vi "Emballge_BDD_Lecture_balises_PPXml_V2.vi"(8 "entrée d'erreur (pas d'erreur)":errorcluster, 11 "appended path":path) -> (0 "sortie d'erreur":errorcluster, 1 "Nb_valve_par_carton":string, 3 "affiche_code_barre_client":string, 4 "melange_des_lots_possible":string, 5 "Code_Barre_Fixe":string, 7 "Indice":string)   [LabVIEW 2020]
uses:
  <vilib>/xml/Load XML File.vi
  <vilib>/xml/Close Reference(Node).vi
  <vilib>/xml/NI_XML.lvlib
panel:
  out "x-y":u32
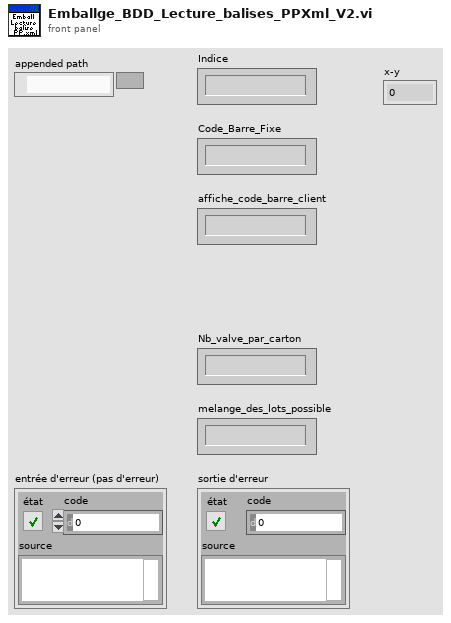
[diagram p1: front panel]
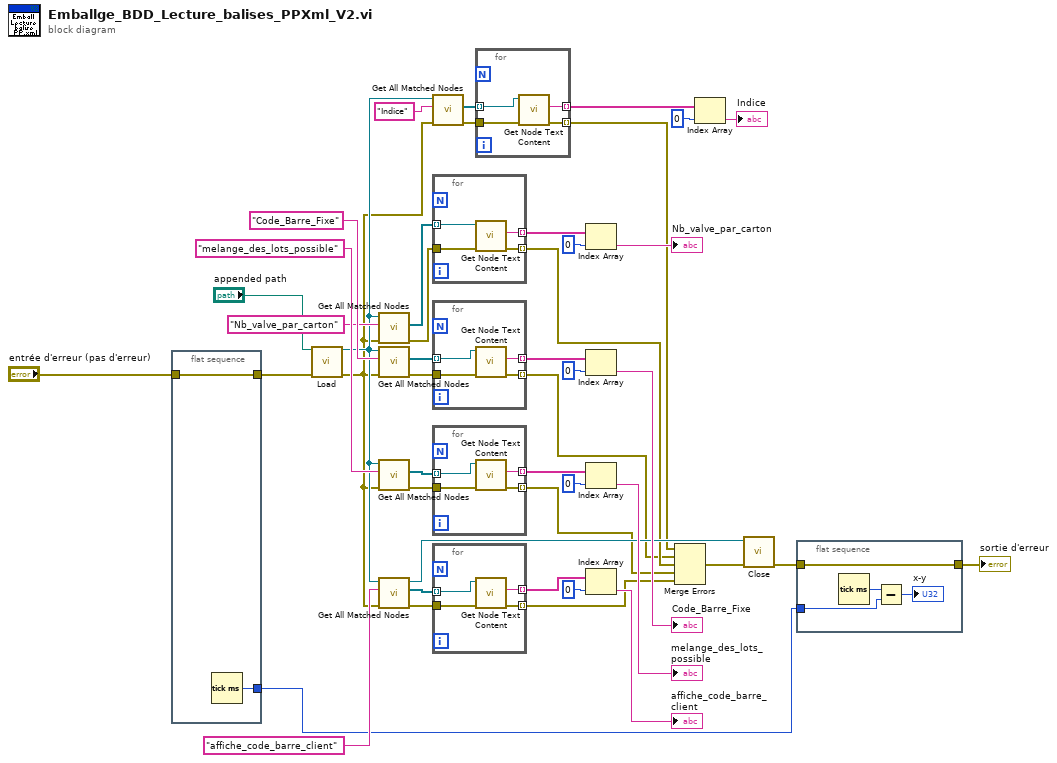
[diagram p0: block diagram]
diagram:
  n1 = flat-sequence {
    tunnel: [w47] -> w33
    tunnel: "entrée d'erreur (pas d'erreur)" -> [w47]
    tunnel: [w46] -> w30
    frame #0 {
      n2 = Tick Count (ms)() -> (millisecond timer value=w46:u32)
    }
  }
  n3 = call-poly <vilib>:"Load.vi"("path to XML document"="appended path", "error in (no error)"=w33) -> ("DOM document out"=w6:refnum<k20>, "error out"=w5:errorcluster)  [unwired: 11 in, 1 out]
  n4 = call <vilib>:"Get All Matched Nodes.vi"("error in (no error)"=w5, "XPath expression"="Nb_valve_par_carton", "node in"=w6) -> ("error out"=w20:errorcluster, "node result array"=w21:refnum<k20>[])  [unwired: 6 in, 1 out]
  n5 = call <vilib>:"Get All Matched Nodes.vi"("error in (no error)"=w5, "XPath expression"="Code_Barre_Fixe", "node in"=w6) -> ("error out"=w24:errorcluster, "node result array"=w25:refnum<k20>[])  [unwired: 6 in, 1 out]
  n6 = call <vilib>:"Get All Matched Nodes.vi"("error in (no error)"=w5, "XPath expression"="melange_des_lots_possible", "node in"=w6) -> ("error out"=w16:errorcluster, "node result array"=w17:refnum<k20>[])  [unwired: 6 in, 1 out]
  n7 = call <vilib>:"Get All Matched Nodes.vi"("error in (no error)"=w5, "XPath expression"="affiche_code_barre_client", "node in"=w6) -> ("error out"=w12:errorcluster, "node result array"=w13:refnum<k20>[], "node out"=w7:refnum<k20>)  [unwired: 6 in]
  n8 = call <vilib>:"Get All Matched Nodes.vi"("error in (no error)"=w5, "XPath expression"="Indice", "node in"=w6) -> ("error out"=w27:errorcluster, "node result array"=w28:refnum<k20>[])  [unwired: 6 in, 1 out]
  n9 = for {
    tunnel: w21 -> [w51] mode=indexing
    tunnel: w20 -> [w50]
    tunnel: [w49] -> w3 mode=indexing
    tunnel: [w48] -> w18 mode=indexing
    n10 = call <vilib>:"Get Node Text Content.vi"("error in (no error)"=w50, "node in"=w51) -> ("error out"=w49:errorcluster, "node text"=w48:string)  [unwired: 7 in, 1 out]
  }
  n11 = for {
    tunnel: w25 -> [w55] mode=indexing
    tunnel: w24 -> [w54]
    tunnel: [w53] -> w2 mode=indexing
    tunnel: [w52] -> w22 mode=indexing
    n12 = call <vilib>:"Get Node Text Content.vi"("error in (no error)"=w54, "node in"=w55) -> ("error out"=w53:errorcluster, "node text"=w52:string)  [unwired: 7 in, 1 out]
  }
  n13 = for {
    tunnel: w17 -> [w59] mode=indexing
    tunnel: w16 -> [w58]
    tunnel: [w57] -> w4 mode=indexing
    tunnel: [w56] -> w14 mode=indexing
    n14 = call <vilib>:"Get Node Text Content.vi"("error in (no error)"=w58, "node in"=w59) -> ("error out"=w57:errorcluster, "node text"=w56:string)  [unwired: 7 in, 1 out]
  }
  n15 = for {
    tunnel: w13 -> [w63] mode=indexing
    tunnel: w12 -> [w62]
    tunnel: [w61] -> w10 mode=indexing
    tunnel: [w60] -> w9 mode=indexing
    n16 = call <vilib>:"Get Node Text Content.vi"("error in (no error)"=w62, "node in"=w63) -> ("error out"=w61:errorcluster, "node text"=w60:string)  [unwired: 7 in, 1 out]
  }
  n17 = for {
    tunnel: w28 -> [w67] mode=indexing
    tunnel: w27 -> [w66]
    tunnel: [w65] -> w1 mode=indexing
    tunnel: [w64] -> w29 mode=indexing
    n18 = call <vilib>:"Get Node Text Content.vi"("error in (no error)"=w66, "node in"=w67) -> ("error out"=w65:errorcluster, "node text"=w64:string)  [unwired: 7 in, 1 out]
  }
  n19 = Index Array(array=w18, index=0 ("indice")) -> (element=→"Nb_valve_par_carton":string)
  n20 = Index Array(array=w22, index=0 ("indice")) -> (element=→"Code_Barre_Fixe":string)
  n21 = Index Array(array=w14, index=0 ("indice")) -> (element=→"melange_des_lots_possible":string)
  n22 = Index Array(array=w9, index=0 ("indice")) -> (element=→"affiche_code_barre_client":string)
  n23 = Merge Errors(w1, w2, w3, w4, w10) -> (w8:errorcluster)
  n24 = Index Array(array=w29, index=0 ("indice")) -> (element=→"Indice":string)
  n25 = call-poly <vilib>:"Close.vi"("error in (no error)"=w8, "node"=w7) -> ("error out"=w32:errorcluster)  [unwired: 7 in]
  n26 = flat-sequence {
    tunnel: [w71] -> w31
    tunnel: w32 -> [w71]
    tunnel: w30 -> [w68]
    frame #0 {
      n27 = Tick Count (ms)() -> (millisecond timer value=w70:u32)
      n28 = Subtract(x=w70, y=w68) -> (x-y=→"x-y":u32)
    }
  }
  "sortie d'erreur" <- w31
